vi "server.Add Response (Custom Error from Request).vi"(4 "message":string, 6 "code":i32, 7 "Request":refnum<class "Request.lvclass">, 8 "error in (no error)":errorcluster, 10 "data":refnum<class "JSON Null.lvclass">, 11 "Server in":refnum<class "JSONRPC Server.lvclass">) -> (0 "error out":errorcluster, 1 "response string":string, 3 "Server out":refnum<class "JSONRPC Server.lvclass">)   [LabVIEW 2016, in "JSONRPC Server.lvclass"]
uses:
  JSONRPC Server.lvclass
  Request/Request.lvclass
  <vilib>/NI/JSON Support for LabVIEW/JSON Data Classes/JSON Datatype/JSON Null.lvclass
  Request/Request.lvclass/Request.ctl
  Request/request.Read jsonrpc.vi
  Request/request.Read id value.vi
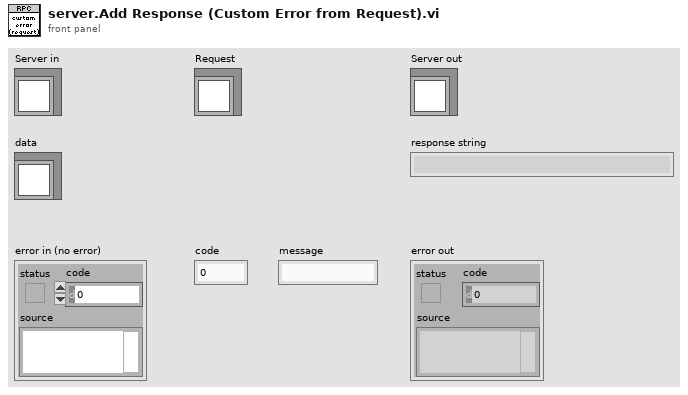
[diagram p1: front panel]
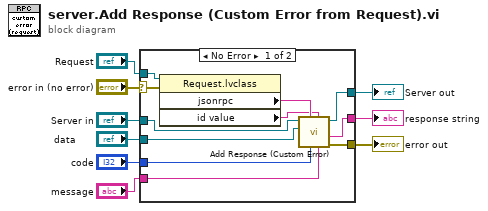
[diagram p0: block diagram]
diagram:
  n1 = case shown="No Error" "error in (no error)" {
    selector: "error in (no error)" -> [w20 w22]
    tunnel: [w11 w22] -> w8
    tunnel: [w12 w21] -> w6
    tunnel: "Server in" -> [w18 w21]
    tunnel: "Request" -> [w19 _]
    tunnel: "code" -> [w16 _]
    tunnel: "message" -> [w15 _]
    tunnel: "data" -> [w17 _]
    tunnel: [w10 _] -> w1
    frame No Error {
      n2 = property class="Request.lvclass"(reference=w19, error in=w20) -> ("jsonrpc"=w14:string, "id value"=w13:string)  [unwired: 2 out]
      n3 = call "Add Response (Custom Error).vi"("message"=w15, "id value"=w13, "code"=w16, "jsonrpc"=w14, "data"=w17, "Server in"=w18) -> ("error out"=w11:errorcluster, "response string"=w10:string, "Server out"=w12:refnum<class "JSONRPC Server.lvclass">)  [unwired: 3 in]
    }
    frame Error {
    }
  }
  "error out" <- w8
  "Server out" <- w6
  "response string" <- w1
